vi "Choreo_Choreo_SwerveController.vi"(6 "Pass_Through_Time":dbl=-1.0 format="%33.4f", 7 "ChoreoSwerveControlConfig":T7={"X_Adv PID Tuning"={"Kf"=0.0, "Kp"=3.0, "Ki"=0.0, "Kd"=0.0, "MaximumIntegral"=9.9e+30, "MinimumIntegral"=-9.9e+30, "Filter Derivative"=FALSE, "IntegralZone"=9.9e+30}, "X_Adv PID Limits"={"MaxInput"=0.0, "MinInput"=0.0, "Continuous"=FALSE, "MaxOutput"=9.9e+32, "MinOutput"=-9.9e+32}, "Y_Adv PID Tuning"={"Kf"=0.0, "Kp"=4.0, "Ki"=0.0, "Kd"=0.0, "MaximumIntegral"=9.9e+30, "MinimumIntegral"=-9.9e+30, "Filter Derivative"=FALSE, "IntegralZone"=9.9e+30}, "Y_Adv PID Limits"={"MaxInput"=0.0, "MinInput"=0.0, "Continuous"=FALSE, "MaxOutput"=9.9e+32, "MinOutput"=-9.9e+32}, "Rot_Adv PID Tuning"={"Kf"=0.0, "Kp"=5.0, "Ki"=0.0, "Kd"=0.0, "MaximumIntegral"=9.9e+30, "MinimumIntegral"=-9.9e+30, "Filter Derivative"=FALSE, "IntegralZone"=9.9e+30}, "Rot_Adv PID Limits"={"MaxInput"=3.141592653589793, "MinInput"=-3.14159, "Continuous"=TRUE, "MaxOutput"=9.9e+32, "MinOutput"=-9.9e+32}, "X Y Pos Tolerance M"=0.0381, "Rot Tolerance Deg"=10.0, "X Y Vel Tolerance M/S"=1.0, "Rot Vel Tolerance Deg/S"=30.0}, 8 "Auto":bool=TRUE, 9 "Reset":bool, 10 "ChoreoSwerveSample":T6, 11 "Current Position":T3={"TRANSLATION"={"X"=0.0, "Y"=0.0}, "ROTATION"={"VALUE"=0.0, "COS"=1.0, "SIN"=0.0}} {"ROTATION"."SIN" format="%13.4f"; "ROTATION"."COS" format="%13.4f"; "ROTATION"."VALUE" format="%13.4f"; "TRANSLATION"."Y" format="%14.3f"; "TRANSLATION"."X" format="%14.3f"}) -> (2 "On Target":bool, 3 "Chassis Speed Dmd":T2 {"vOmega" format="%10.3f"; "vY" format="%10.3f"; "vX" format="%10.3f"}, 4 "Ctrl Info":T1)   [LabVIEW 2019, in "ChoreoLib.lvlib"]
doc: "Creates and executes a swerve drive control function to execute a Choreo Trajectory sample. The controller consists of three advanced PID controllers, one for X position, Y position, and Rotation.\n\nInputs:\n - ChoreoSwerveControlConfig - cluster - Controller configuration data\n - Current Pose - pose2d - Current robot position pose calcualted by either Odometry or Pose Estimation.\n - ChoreoTrajectoryState - cluster - Trajectory state to execute\n - Reset - boolean - Resets the controllers.\n - Auto - boolean - When TRUE closed loop control is used to control trajectory execution. This is mostly for debugging and robot tuning. (Optional. Default: TRUE )\n - PassThroughTime - double - Continueually counting time (seconds) read from the FGPA on roboRIO or local computer when running on PC. (Optional: Default: Read FGPA time )\n\nOutputs:\n - Choreo Speed Demand - chassis speed - Desired chassis speed (M/S, Rad/Sec)\n - On Target - boolean - TRUE when robot position is within tolerance of trajectory position\n - Ctrl Info - cluster - Information on control. Mostly for diagnostics."
uses:
  ChoreoLib.lvlib
  TypeDef/ChoreoSwerveControlConfig.ctl
  <vilib>/Rock Robotics/WPI/ThirdParty/JAS_Junk/TrajLib/TypeDef/PID_ADV_TUNING.ctl
  <vilib>/Rock Robotics/WPI/ThirdParty/JAS_Junk/TrajLib/TypeDef/PID_ADV_LIMITS.ctl
  <vilib>/Rock Robotics/WPI/ThirdParty/JAS_Junk/TrajLib/TypeDef/POSE2D.ctl
  <vilib>/Rock Robotics/WPI/ThirdParty/JAS_Junk/TrajLib/TypeDef/TRANSLATION2D.ctl
  <vilib>/Rock Robotics/WPI/ThirdParty/JAS_Junk/TrajLib/TypeDef/ROTATION2D.ctl
  <vilib>/Rock Robotics/WPI/ThirdParty/JAS_Junk/TrajLib/TypeDef/CHASSIS_SPEEDS.ctl
  <vilib>/Rock Robotics/WPI/ThirdParty/JAS_Junk/TrajLib/TypeDef/PID_ERROR_TOLERANCE.ctl
  <vilib>/Rock Robotics/WPI/ThirdParty/JAS_Junk/TrajLib/VI/Util_GetTime_U32.vi
  <vilib>/Rock Robotics/WPI/ThirdParty/JAS_Junk/TrajLib/PIDController_AtSetpoint.vi
  <vilib>/Rock Robotics/WPI/ThirdParty/JAS_Junk/TrajLib/PIDController_SetPIDF.vi
  <vilib>/Rock Robotics/WPI/ThirdParty/JAS_Junk/TrajLib/PIDController_SetDerivativeFilter.vi
  <vilib>/Rock Robotics/WPI/ThirdParty/JAS_Junk/TrajLib/PIDController_SetIntegratorRange.vi
  <vilib>/Rock Robotics/WPI/ThirdParty/JAS_Junk/TrajLib/PIDController_SetTolerancePandV.vi
  <vilib>/Rock Robotics/WPI/ThirdParty/JAS_Junk/TrajLib/PIDController_DisableContinousInput.vi
  <vilib>/Rock Robotics/WPI/ThirdParty/JAS_Junk/TrajLib/PIDController_EnableContinousInput.vi
  <vilib>/Rock Robotics/WPI/ThirdParty/JAS_Junk/TrajLib/PIDController_Reset.vi
  <vilib>/Rock Robotics/WPI/ThirdParty/JAS_Junk/TrajLib/PIDController_New.vi
  <vilib>/Rock Robotics/WPI/ThirdParty/JAS_Junk/TrajLib/PIDController_SetOutputLimits.vi
  <vilib>/Rock Robotics/WPI/ThirdParty/JAS_Junk/TrajLib/VI/PIDController_SetIntegratorZone.vi
  <vilib>/Rock Robotics/WPI/ThirdParty/JAS_Junk/TrajLib/Rotation2d_GetCos.vi
  <vilib>/Rock Robotics/WPI/ThirdParty/JAS_Junk/TrajLib/Rotation2d_GetSin.vi
  <vilib>/Rock Robotics/WPI/ThirdParty/JAS_Junk/TrajLib/ChassisSpeeds_New.vi
  <vilib>/Rock Robotics/WPI/ThirdParty/JAS_Junk/TrajLib/PIDController_NewPeriod.vi
  <vilib>/Rock Robotics/SystemInterfaces/NetworkCommunication/NetComm_UsageReport_report.vi
  <vilib>/Rock Robotics/WPI/ThirdParty/JAS_Junk/TrajLib/VI/Util_GetTime_U64.vi
  <vilib>/Rock Robotics/WPI/ThirdParty/JAS_Junk/TrajLib/Globals/Util_LibraryGlobals.vi
  <vilib>/Rock Robotics/WPI/ThirdParty/JAS_Junk/TrajLib/PIDController_AdvCalculate_FF_Sp_Pv.vi
  <vilib>/Rock Robotics/WPI/ThirdParty/JAS_Junk/TrajLib/Trajectory_Library.lvlib
  TypeDef/ChoreoSwerveSample.ctl
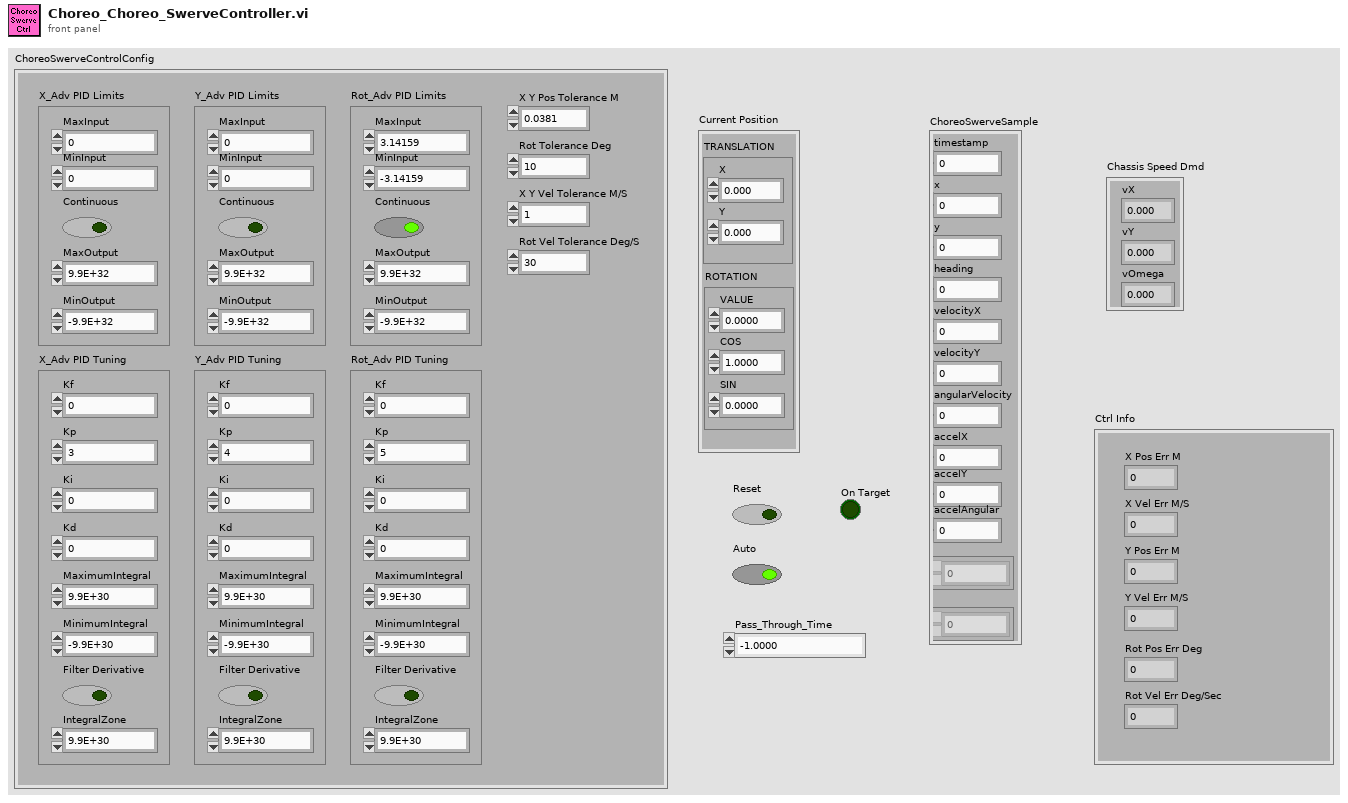
[diagram p1: front panel]
types:
  T1 = cluster{"X Pos Err M":dbl, "X Vel Err M/S":dbl, "Y Pos Err M":dbl, "Y Vel Err M/S":dbl, "Rot Pos Err Deg":dbl, "Rot Vel Err Deg/Sec":dbl}
  T2 = typedef "Trajectory_Library.lvlib/CHASSIS_SPEEDS.ctl" = cluster{"vX":dbl, "vY":dbl, "vOmega":dbl}
  T3 = typedef "Trajectory_Library.lvlib/POSE2D.ctl" = cluster{"TRANSLATION":T4, "ROTATION":T5}
  T4 = typedef "Trajectory_Library.lvlib/TRANSLATION2D.ctl" = cluster{"X":dbl, "Y":dbl}
  T5 = typedef "Trajectory_Library.lvlib/ROTATION2D.ctl" = cluster{"VALUE":dbl, "COS":dbl, "SIN":dbl}
  T6 = typedef "ChoreoLib.lvlib/ChoreoSwerveSample.ctl" = cluster{"timestamp":dbl, "x":dbl, "y":dbl, "heading":dbl, "velocityX":dbl, "velocityY":dbl, "angularVelocity":dbl, "accelX":dbl, "accelY":dbl, "accelAngular":dbl, "forceX":dbl[], "forceY":dbl[]}
  T7 = typedef "ChoreoLib.lvlib/ChoreoSwerveControlConfig.ctl" = cluster{"X_Adv PID Tuning":T8, "X_Adv PID Limits":T9, "Y_Adv PID Tuning":T8, "Y_Adv PID Limits":T9, "Rot_Adv PID Tuning":T8, "Rot_Adv PID Limits":T9, "X Y Pos Tolerance M":dbl, "Rot Tolerance Deg":dbl, "X Y Vel Tolerance M/S":dbl, "Rot Vel Tolerance Deg/S":dbl}
  T8 = typedef "Trajectory_Library.lvlib/PID_ADV_TUNING.ctl" = cluster{"Kf":dbl, "Kp":dbl, "Ki":dbl, "Kd":dbl, "MaximumIntegral":dbl, "MinimumIntegral":dbl, "Filter Derivative":bool, "IntegralZone":dbl}
  T9 = typedef "Trajectory_Library.lvlib/PID_ADV_LIMITS.ctl" = cluster{"MaxInput":dbl, "MinInput":dbl, "Continuous":bool, "MaxOutput":dbl, "MinOutput":dbl}
  T10 = typedef "Trajectory_Library.lvlib/PID_ERROR_TOLERANCE.ctl" = cluster{"PositionTolerance":dbl, "VelocityTolerance":dbl}
  T11 = typedef "Trajectory_Library.lvlib/PID_CONTROLLER.ctl" = cluster{"Kp":dbl, "Ki":dbl, "Kd":dbl, "Period":dbl, "Max_Integral":dbl, "Min_Integral":dbl, "Max_Input":dbl, "Min_Input":dbl, "Continuous":bool, "PositionError":dbl, "VelocityError":dbl, "PrevError":dbl, "Total_Integral":dbl, "PositionTolerance":dbl, "VelocityTolerance":dbl, "SetPoint":dbl, "Kf":dbl, "Prev_Deriv":dbl, "Prev_Deriv 2":dbl, "DerivativeFilter":bool, "Min_Output":dbl, "Max_Output":dbl, "Prev_F_P":dbl, "Prev_F_P_2":dbl, "AntiWindupActive":bool, "Measurement":dbl, "IntegralZone":dbl}
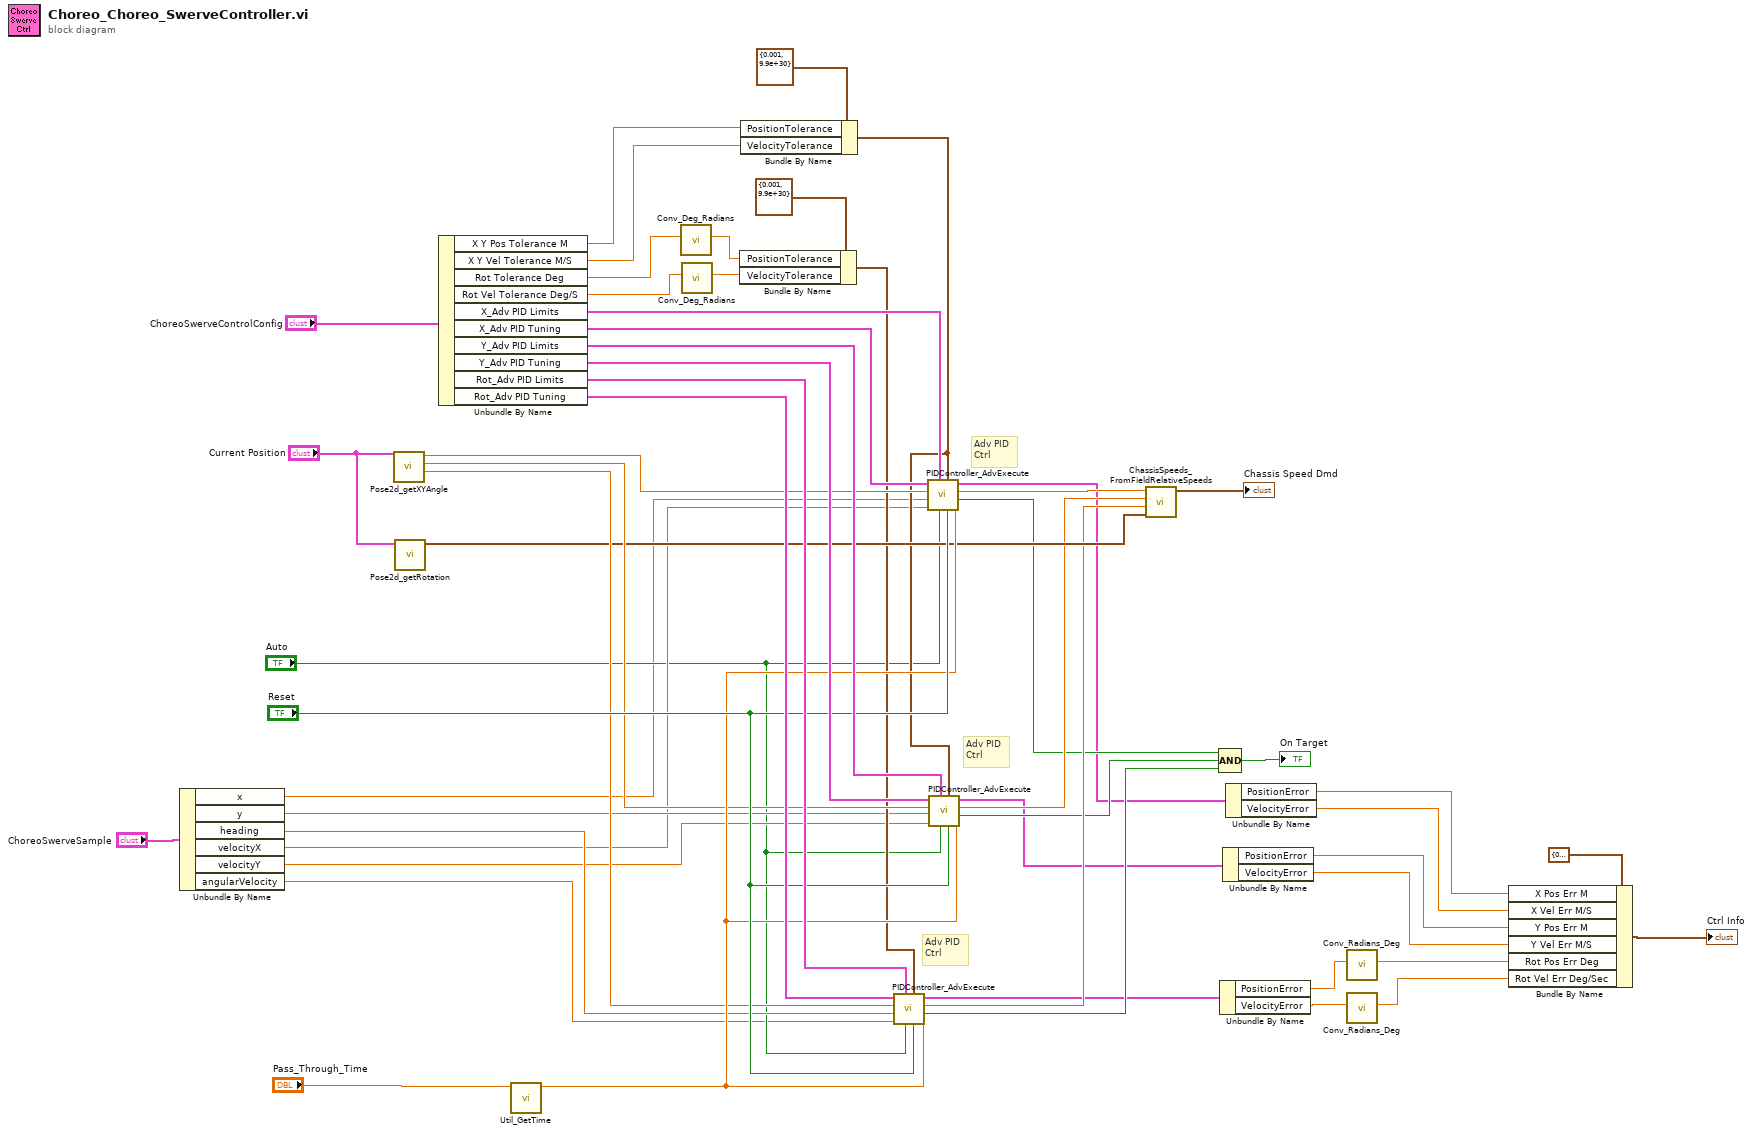
[diagram p0: block diagram]
diagram:
  # "Adv PID\nCtrl"
  # "Adv PID\nCtrl"
  # "Adv PID\nCtrl"
  n1 = Unbundle By Name("ChoreoSwerveSample") -> ("x"=w1:dbl, "y"=w7:dbl, "heading"=w6:dbl, "velocityX"=w5:dbl, "velocityY"=w4:dbl, "angularVelocity"=w2:dbl)
  n2 = call <vilib>:"Pose2d_getXYAngle.vi"("in POSE"="Current Position") -> ("Angle"=w42:dbl, "Y"=w43:dbl, "X"=w44:dbl)  [unwired: 8 in]
  n3 = call <vilib>:"Pose2d_getRotation.vi"("in POSE"="Current Position") -> ("out ROTATION"=w40:T5)  [unwired: 10 in]
  n4 = Unbundle By Name("ChoreoSwerveControlConfig") -> ("X Y Pos Tolerance M"=w28:dbl, "X Y Vel Tolerance M/S"=w27:dbl, "Rot Tolerance Deg"=w12:dbl, "Rot Vel Tolerance Deg/S"=w11:dbl, "X_Adv PID Limits"=w54:T9, "X_Adv PID Tuning"=w53:T8, "Y_Adv PID Limits"=w52:T9, "Y_Adv PID Tuning"=w51:T8, "Rot_Adv PID Limits"=w50:T9, "Rot_Adv PID Tuning"=w49:T8)
  n5 = call <vilib>:"Util_GetTime.vi"("Pass_Through_Time"="Pass_Through_Time") -> ("FPGA_Time_Seconds"=w46:dbl)  [unwired: 8 in, 2 out]
  n6 = call <vilib>:"Conv_Deg_Radians.vi"("Degress"=w12) -> ("Radians"=w9:dbl)  [unwired: 10 in]
  n7 = call <vilib>:"Conv_Deg_Radians.vi"("Degress"=w11) -> ("Radians"=w10:dbl)  [unwired: 10 in]
  n8 = Bundle By Name(cluster=T10 {"PositionTolerance"=0.001, "VelocityTolerance"=9.9e+30} ("PID Error Tolerance"), "PositionTolerance"=w9, "VelocityTolerance"=w10) -> (w26:T10)
  n9 = Bundle By Name(cluster=T10 {"PositionTolerance"=0.001, "VelocityTolerance"=9.9e+30} ("PID Error Tolerance"), "PositionTolerance"=w28, "VelocityTolerance"=w27) -> (w30:T10)
  n10 = call <vilib>:"PIDController_AdvExecute.vi"("Time"=w46, "Reset"="Reset", "PID Error Tolerance"=w26, "Auto"="Auto", "Adv PID Limits"=w50, "FF-FeedForward"=w2, "SP-SetPoint"=w6, "PV-Measurement"=w42, "Adv PID Tuning"=w49) -> ("AtSetpoint"=w33:bool, "CO-ControlOutput"=w37:dbl, "out PID_CONTROLLER"=w21:T11)
  n11 = call <vilib>:"PIDController_AdvExecute.vi"("Time"=w46, "Reset"="Reset", "PID Error Tolerance"=w30, "Auto"="Auto", "Adv PID Limits"=w54, "FF-FeedForward"=w5, "SP-SetPoint"=w1, "PV-Measurement"=w44, "Adv PID Tuning"=w53) -> ("AtSetpoint"=w35:bool, "CO-ControlOutput"=w39:dbl, "out PID_CONTROLLER"=w25:T11)
  n12 = call <vilib>:"PIDController_AdvExecute.vi"("Time"=w46, "Reset"="Reset", "PID Error Tolerance"=w30, "Auto"="Auto", "Adv PID Limits"=w52, "FF-FeedForward"=w4, "SP-SetPoint"=w7, "PV-Measurement"=w43, "Adv PID Tuning"=w51) -> ("AtSetpoint"=w34:bool, "CO-ControlOutput"=w38:dbl, "out PID_CONTROLLER"=w22:T11)
  n13 = call <vilib>:"ChassisSpeeds_FromFieldRelativeSpeeds.vi"("RobotAngle"=w40, "Omega"=w37, "vY"=w38, "vX"=w39) -> ("CHASSIS"=→"Chassis Speed Dmd":T2)  [unwired: 7 in]
  n14 = Compound Arithmetic op=AND(w35, w34, w33) -> (→"On Target":bool)
  n15 = Unbundle By Name(w21) -> ("PositionError"=w16:dbl, "VelocityError"=w15:dbl)
  n16 = Unbundle By Name(w22) -> ("PositionError"=w18:dbl, "VelocityError"=w17:dbl)
  n17 = Unbundle By Name(w25) -> ("PositionError"=w20:dbl, "VelocityError"=w19:dbl)
  n18 = call <vilib>:"Conv_Radians_Deg.vi"("Radians"=w16) -> ("Degrees"=w14:dbl)  [unwired: 10 in]
  n19 = call <vilib>:"Conv_Radians_Deg.vi"("Radians"=w15) -> ("Degrees"=w13:dbl)  [unwired: 10 in]
  n20 = Bundle By Name(cluster=T1 {"X Pos Err M"=0.0, "X Vel Err M/S"=0.0, "Y Pos Err M"=0.0, "Y Vel Err M/S"=0.0, "Rot Pos Err Deg"=0.0, "Rot Vel Err Deg/Sec"=0.0} ("Info"), "X Pos Err M"=w20, "X Vel Err M/S"=w19, "Y Pos Err M"=w18, "Y Vel Err M/S"=w17, "Rot Pos Err Deg"=w14, "Rot Vel Err Deg/Sec"=w13) -> (→"Ctrl Info":T1)
